vi "subLogin.vi"(4 "Login Button":bool, 6 "Password Entry":string, 7 "Password Array":string[](array[string]), 8 "User Entry":string, 9 "User Array":string[](array[string])) -> (0 "Array Index No":i32, 1 "If Correct 2":bool, 2 "If Correct 1":bool, 3 "If Incorrect":bool, 5 "Username Out":string)   [LabVIEW 2017]
panel:
  # "This VI checks two user entered string values\nagainst two pre-created arrays to check that the\nindex elements are the same and match.\nIf not, it outputs true to \"If Correct\" and -1 to\nIndex No when Login is pressed, otherwise it outputs\nthe array Index number and two true outputs to\nIf Correct 1 and 2."
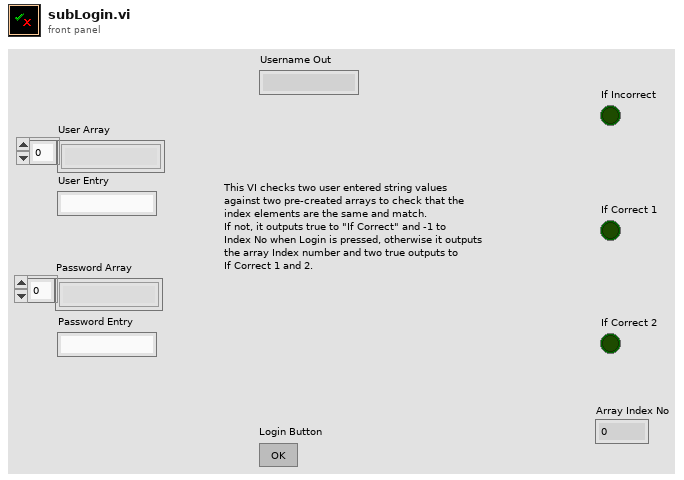
[diagram p1: front panel]
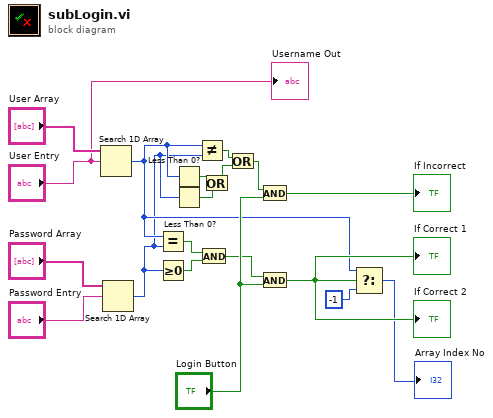
[diagram p0: block diagram]
diagram:
  n1 = Search 1D Array(1D array="User Array", element="User Entry") -> (index of element=w3:i32)  [unwired: 1 in]
  n2 = Search 1D Array(1D array="Password Array", element="Password Entry") -> (index of element=w2:i32)  [unwired: 1 in]
  n3 = Equal?(x=w3, y=w2) -> (x = y?=w16:bool)
  n4 = Greater Or Equal To 0?(x=w2) -> (x >= 0?=w17:bool)
  n5 = Less Than 0?(x=w3) -> (x < 0?=w6:bool)
  n6 = Less Than 0?(x=w2) -> (x < 0?=w5:bool)
  n7 = Not Equal?(x=w3, y=w2) -> (x != y?=w7:bool)
  n8 = And(x=w16, y=w17) -> (x .and. y?=w18:bool)
  n9 = Or(x=w6, y=w5) -> (x .or. y?=w4:bool)
  n10 = Or(x=w7, y=w4) -> (x .or. y?=w1:bool)
  n11 = And(x=w1, y="Login Button") -> (x .and. y?=→"If Incorrect":bool)
  n12 = And(x=w18, y="Login Button") -> (x .and. y?=w9:bool)
  "If Correct 1" <- w9
  "If Correct 2" <- w9
  n13 = Select(t=w3, s=w9, f=-1) -> (s? t:f=→"Array Index No":i32)
  "Username Out" <- "User Entry"
